vi "Main.vi"(8 "error in (no error)":errorcluster, 11 "Logging Thread in":refnum<class "Logging Thread.lvclass">) -> (0 "error out":errorcluster, 3 "Logging Thread out":refnum<class "Logging Thread.lvclass">)   [LabVIEW 2019, in "DSF Core.lvlib" / "Logging Thread.lvclass"]
uses:
  Logging Thread.lvclass
  C:/Dev/GitHub/niveristand-data-sharing-framework-custom-device/Core/Classes/Thread/Thread.lvclass
  Logging Thread.lvclass/Logging Thread.ctl
  Interface/Interface.lvclass/Interface.ctl
  Pointers/Error/Error Pointer.lvclass/Error Pointer.ctl
  <vilib>/NI/Memory Manager/Classes/Pointer/Pointer.lvclass/Pointer.ctl
  Thread.lvclass/Thread.ctl
  Interface/Logging/Wait For.vi
  Interface/Logging/Wait For Logging Command.vi
  Interface/Logging/Send.vi
  Interface/Logging/Send Logging Response.vi
  Pointers/Error/Read Error Pointer.vi
  Pointers/Error/Encapsulate Error.vi
  Get Plugin Thread Name.vi
  <vilib>/NI/Memory Manager/Classes/Pointer/Write.vi
  <vilib>/NI/Memory Manager/Classes/Pointer/Write Bool.vi
  <vilib>/NI/Memory Manager/Classes/Pointer/Read.vi
  <vilib>/NI/Memory Manager/Classes/Pointer/Read Bool.vi
  Close Log File.vi
  <vilib>/Utility/High Resolution Relative Seconds.vi
  Write Log File.vi
  Interface/Errors.vi
  Interface/Dispatcher/Command Timeout.vi
  Interface/Send Response.vi
  Interface/Dispatcher/Response Timeout.vi
  <vilib>/Utility/error.llb/Clear Errors.vi
  <vilib>/NI/Memory Manager/Classes/Pointer/Read 1D U8.vi
  Trim Error Whitespace.vi
  Pointers/Error/Get Power Of 2.vi
  <vilib>/NI/Memory Manager/Classes/Pointer/Encapsulate.vi
  Pointers/Error/Error Size.vi
  <vilib>/NI/Memory Manager/Classes/Pointer/Write (No Check).vi
  <vilib>/NI/Memory Manager/Classes/Pointer/Write (No Check) Bool.vi
  <vilib>/NI/Memory Manager/Classes/Pointer/Check Move.vi
  <vilib>/NI/Memory Manager/Classes/Pointer/Read (No Check).vi
  <vilib>/NI/Memory Manager/Classes/Pointer/Read (No Check) Bool.vi
  Interface/Read RT FIFO.vi
  Interface/New Interface Error.vi
  Interface/Write RT FIFO.vi
  <vilib>/NI/Memory Manager/Classes/Pointer/Read (No Check) 1D U8.vi
  <vilib>/NI/Memory Manager/Classes/Pointer/Set Size.vi
  <vilib>/NI/Memory Manager/Classes/Pointer/Set Address.vi
  <vilib>/NI/Memory Manager/Classes/Pointer/Check Null Pointer.vi
  <vilib>/NI/Memory Manager/Classes/Pointer/Set Internal.vi
  <vilib>/NI/Memory Manager/Classes/Pointer/Get Address.vi
  <vilib>/NI/Memory Manager/Classes/Pointer/Check Count.vi
  <vilib>/NI/Memory Manager/Classes/Pointer/Check Bounds (Power of 2).vi
  <vilib>/NI/Memory Manager/VIs/New Error Cluster.vi
  <vilib>/NI/Memory Manager/VIs/New Error Cluster (512B).vi
  <vilib>/NI/Memory Manager/VIs/Set Error Code.vi
  <vilib>/NI/Memory Manager/VIs/Set Error Status.vi
  <vilib>/NI/Memory Manager/VIs/Set Error Source.vi
  <vilib>/NI/Memory Manager/VIs/Write String to Source.vi
  Interface/Interface Error Info.vi
  <vilib>/NI/Memory Manager/Classes/Pointer/Errors.vi
  <vilib>/NI/Memory Manager/Classes/Pointer/Null Pointer.vi
  <vilib>/NI/Memory Manager/Classes/Pointer/Is Null.vi
  <vilib>/NI/Memory Manager/Classes/Pointer/Get Size.vi
  <vilib>/NI/Memory Manager/Classes/Pointer/Out of Bounds.vi
  <vilib>/NI/Memory Manager/Classes/Pointer/Check Bounds.vi
  VIs/Constants/Constants.vi
  VIs/Constants/Base Error Code.vi
  Interface/Interface Error Offset.vi
  <vilib>/NI/Memory Manager/Classes/Pointer/Create Error.vi
  <vilib>/NI/Memory Manager/Classes/Pointer/Write Pointer Size to Error.vi
  <vilib>/NI/Memory Manager/VIs/Write Numeric to Source.vi
  <vilib>/NI/Memory Manager/VIs/Write Numeric Scalar to Source (Base10 U64).vi
  <vilib>/NI/Memory Manager/Classes/Pointer/Check Bounds (Pointer).vi
  <vilib>/NI/Memory Manager/Classes/Pointer/Check Bounds (Buffer).vi
  <vilib>/NI/Memory Manager/Constants/Constants.vi
  <vilib>/NI/Memory Manager/Constants/Library Name.vi
  <vilib>/NI/Memory Manager/Classes/Pointer/Pointer Error Info.vi
  <vilib>/NI/Memory Manager/Constants/Pointer Class Name.vi
  <vilib>/NI/Memory Manager/Classes/Pointer/Buffer Underflow.vi
  Interface/Logging/Logging Interface.lvclass
  C:/Dev/GitHub/niveristand-data-sharing-framework-custom-device/Core/Classes/Interface/Interface.lvclass
  Pointers/Error/Error Pointer.lvclass
  C:/Program Files (x86)/National Instruments/LabVIEW 2019/vi.lib/NI/Memory Manager/Classes/Pointer/Pointer.lvclass
  VIs/VI Name.vi
  Thread.lvclass
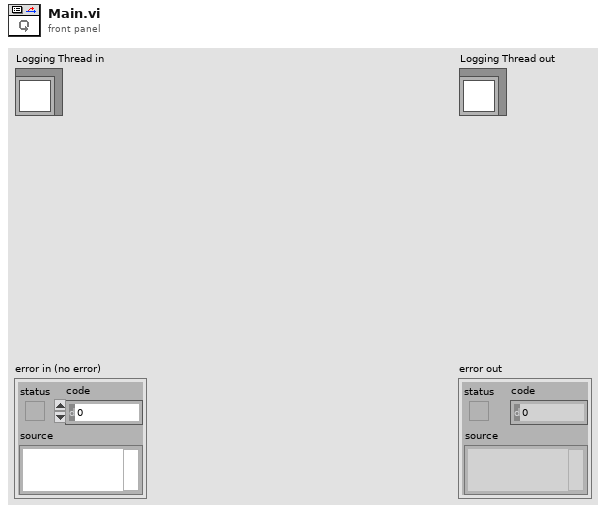
[diagram p1: front panel]
types:
  T1 = typedef "DSF Core.lvlib/Logging Interface.lvclass/Command Data.ctl" = cluster{"Command":T2, "Parameters":T3}
  T2 = typedef "DSF Core.lvlib/Logging Interface.lvclass/Command.ctl" = enum8{"Idle", "Start", "Log Framework State", "Log Plugin State", "Log Dispatcher State", "Shutdown"}
  T3 = typedef "DSF Core.lvlib/Logging Interface.lvclass/Parameters.ctl" = cluster{"arg1":u64, "arg2":u64}
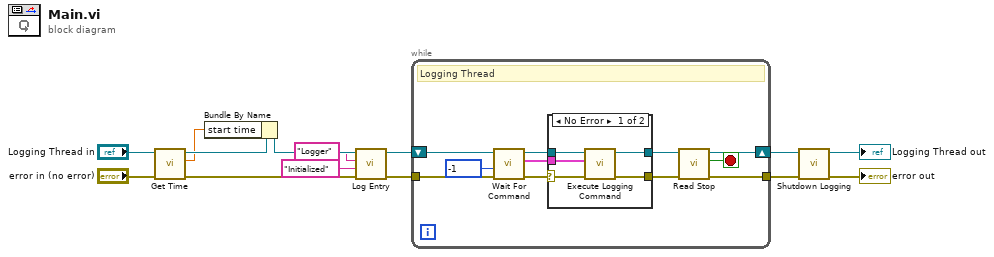
[diagram p0: block diagram]
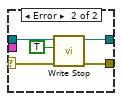
[diagram p2: hidden frame]
diagram:
  n1 = call "Get Time.vi"("error in (no error)"="error in (no error)", "Logging Thread in"="Logging Thread in") -> ("error out"=w3:errorcluster, "time"=w7:dbl, "Logging Thread out"=w8:refnum<class "Logging Thread.lvclass">)  [unwired: 7 in]
  n2 = Bundle By Name(cluster=w8, "start time"=w7) -> (w5:refnum<class "Logging Thread.lvclass">)
  n3 = call "Log Entry.vi"("error in (no error)"=w3, "line text"="Initialized", "line tag"="Logger", "Logging Thread in"=w5) -> ("error out"=w2:errorcluster, "Logging Thread out"=w4:refnum<class "Logging Thread.lvclass">)  [unwired: 6 in]
  n4 = while {
    tunnel: w2 -> [w25]
    tunnel: [w17] -> w13
    shift-right: [w18] -> w14
    shift-left: w4 -> [w24]
    stop <- w16 stop-if-true
    # "Logging Thread"
    n5 = call "Wait For Command.vi"("error in (no error)"=w25, "timeout in ms (0)"=-1, "Logging Thread in"=w24) -> ("error out"=w23:errorcluster, "command"=w15:T1, "Logging Thread out"=w22:refnum<class "Logging Thread.lvclass">)  [unwired: 6 in]
    n6 = case shown="No Error" w23 {
      selector: w23 -> [w30 w33]
      tunnel: [w26 w31] -> w19
      tunnel: w22 -> [w29 w34]
      tunnel: [w27 w32] -> w20
      tunnel: w15 -> [w28 _]
      frame No Error {
        n7 = call "Execute Logging Command.vi"("error in (no error)"=w30, "command"=w28, "Logging Thread in"=w29) -> ("error out"=w26:errorcluster, "Logging Thread out"=w27:refnum<class "Logging Thread.lvclass">)  [unwired: 7 in]
      }
      frame Error {
        n8 = call "Write Stop.vi"("error in (no error)"=w33, "stop"=TRUE, "Thread in"=w34) -> ("error out"=w31:errorcluster, "Thread out"=w32:refnum<class "Logging Thread.lvclass">)  [unwired: 7 in]
      }
    }
    n9 = call "Read Stop.vi"("error in (no error)"=w19, "Thread in"=w20) -> ("error out"=w17:errorcluster, "stop"=w16:bool, "Thread out"=w18:refnum<class "Logging Thread.lvclass">)  [unwired: 7 in]
  }
  n10 = call "Shutdown Logging.vi"("error in (no error)"=w13, "Logging Thread in"=w14) -> ("error out"=→"error out":errorcluster, "Logging Thread out"=→"Logging Thread out":refnum<class "Logging Thread.lvclass">)  [unwired: 8 in]
